vi "PID Values.vi"() -> ()   [LabVIEW 2018]
panel:
  in  "Climber Pivot PID 2":T1={"P"=0.4, "I"=0.0, "D"=0.0, "F"=0.0, "I Zone"=0.0}
  in  "Elevator PID":T1={"P"=0.7, "I"=0.0, "D"=0.05, "F"=0.0, "I Zone"=0.0}
  in  "Shooter Pivot":T1={"P"=0.6, "I"=0.0, "D"=0.0, "F"=0.0, "I Zone"=0.0}
  in  "Climber Pivot PID":T1={"P"=0.3, "I"=0.0, "D"=0.0, "F"=0.0, "I Zone"=0.0}
  # "PID settings for CAN Talon SRX controllers.\nWhen changing, remember to make new values default."
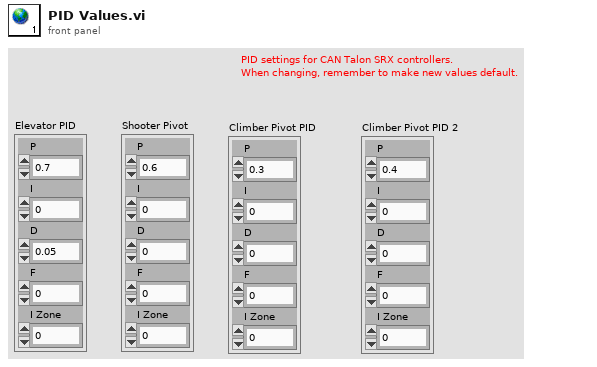
[diagram p1: front panel]
types:
  T1 = cluster{"P":dbl, "I":dbl, "D":dbl, "F":dbl, "I Zone":dbl}
diagram:
